vi "Labview online.vi"() -> ()   [LabVIEW 2019]
uses:
  <vilib>/sound2/lvsound2.llb/Sound Data Format.ctl
  <vilib>/sound2/lvsound2.llb/Sampling Mode.ctl
  <vilib>/sound2/lvsound2.llb/Sound Input Read (DBL).vi
  <vilib>/sound2/lvsound2.llb/Sound Output Write (DBL).vi
  <vilib>/Analysis/NI_AAL_SigProc.lvlib
  <vilib>/gmath/NI_Gmath.lvlib
panel:
  out "Envelope do Sinal":dynamicdata(graph)
  in  "stop":bool
  in  "Email":string
  in  "Gravar e Enviar":bool
  in  "Som de Saída":path
  in  "Terminar Medição":bool
  out "Número de Amostras Totais":dbl
  out "Taxa de Amostragem do Microfone (S/s)":dbl
  in  "Sound Format Input":T1={"sample rate (S/s)"=22050.0, "number of channels"=2, "bits per sample"=16}
  out "Ritmo Cardíaco Médio":dbl format="%0.2f"
  in  "Classificação do Ritmo Cardíaco":bool
  out "Taquicardia":bool
  out "Ritmo Cardíaco Normal":bool
  out "Bradicardia":bool
  in  "Continuar":bool
  out "Sinal Amplificado":waveform(dbl)[](graph)
  out "Sinal Amplificado e Filtrado":dynamicdata(graph)
  in  "Pulmões  ou Coração (pressionar)":bool
  in  "Controlador de Threshold":dbl(slide) scale=0.0..0.01
  out "Ritmo Cardíaco Instantaneo":dbl
  out "Offline Sound":dbl[](array[numeric])
  # "Estetoscópio Digital"
  # "Resultados"
  # "Configurações e Controlos"
  # "Parâmetros do Sinal de Som"
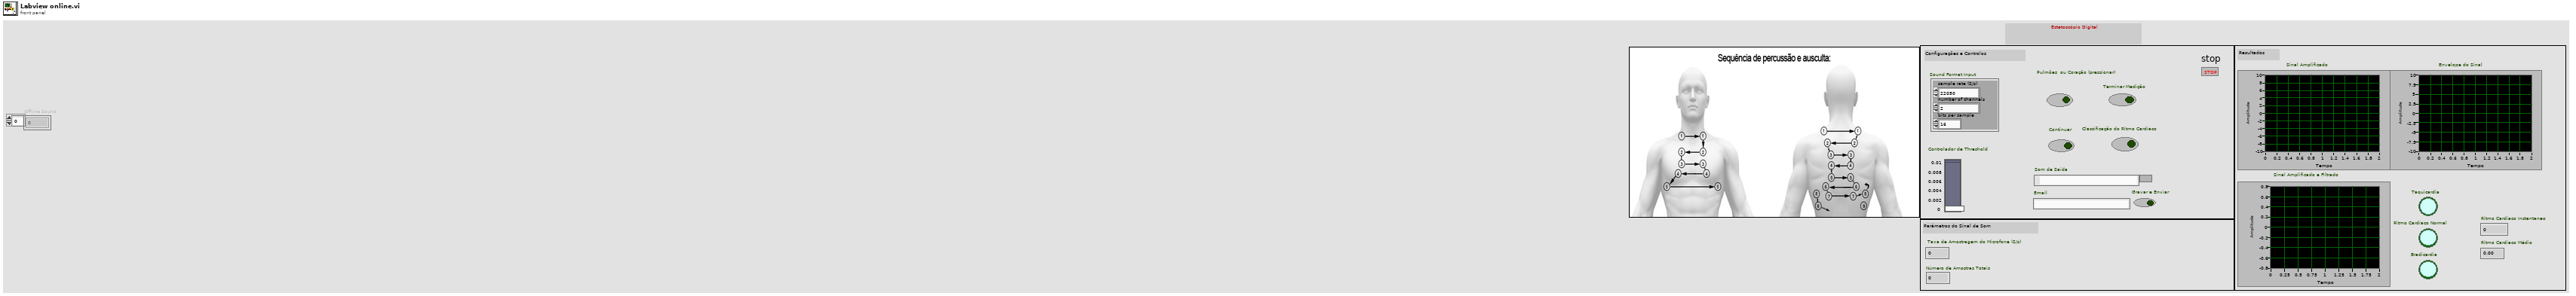
[diagram p1: front panel]
types:
  T1 = typedef "Sound Data Format.ctl" = cluster{"sample rate (S/s)":dbl, "number of channels":i32, "bits per sample":i32}
  T2 = typedef "Sampling Mode.ctl" = i32
  T3 = typedef "Sound Output Task ID.ctl" = u32
  T4 = typedef "Sound Input Task ID.ctl" = u32
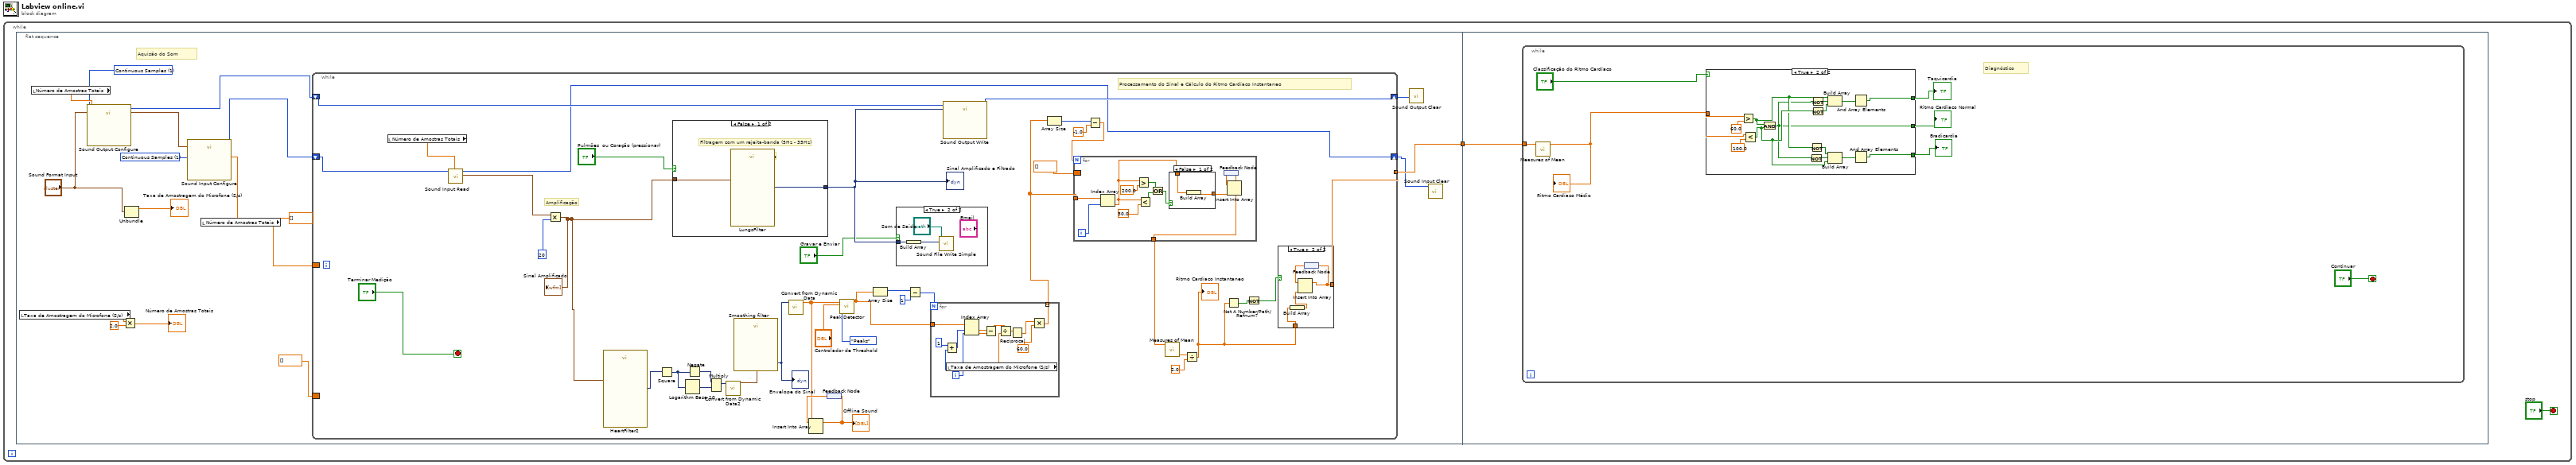
[diagram p0: block diagram]
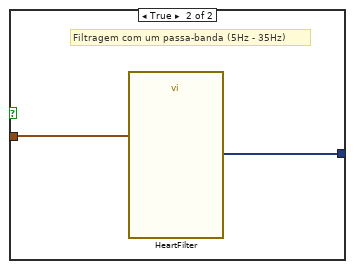
[diagram p5: hidden frame]
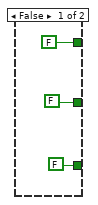
[diagram p6: hidden frame]
diagram:
  n1 = while {
    stop <- "stop" stop-if-true
    n2 = flat-sequence {
      tunnel: [w15] -> w2
      tunnel: w2 -> [w95]
      frame #0 {
        w6 = T2 1 items=["Finite Samples", "Continuous Samples"] ("sample mode")
        w14 = T2 1 items=["Finite Samples", "Continuous Samples"] ("sample mode")
        # "Aquisão do Som"
        n3 = local read "Taxa de Amostragem do Microfone (S/s)"() -> (w11:dbl)
        n4 = local read "Número de Amostras Totais"() -> (w8:dbl)
        n5 = call <vilib>:"Sound Output Configure.vi"("number of samples/ch"=w8, "sample mode"=w6, "sound format"="Sound Format Input") -> ("task ID"=w3:T3)  [unwired: 3 in, 5 out]
        n6 = Multiply(x=w11, y=2.0) -> (x*y=→"Número de Amostras Totais":dbl)
        n7 = Unbundle("Sound Format Input") -> ("sample rate (S/s)"=→"Taxa de Amostragem do Microfone (S/s)":dbl)  [unwired: 2 out]
        n8 = local read "Número de Amostras Totais"() -> (w7:dbl)
        n9 = call <vilib>:"Sound Input Configure.vi"("number of samples/ch"=w7, "sample mode"=w14, "sound format"="Sound Format Input") -> ("task ID"=w5:T4)  [unwired: 3 in, 5 out]
        n10 = while {
          shift-right: [w57] -> w16
          shift-left: w3 -> [w28]
          tunnel: [w44] -> w15
          border: dbl[] [] -> [_]
          border: dbl[] [] -> [_]
          shift-right: [w24] -> w4
          shift-left: w5 -> [w26]
          stop <- "Terminar Medição" stop-if-true
          # "Processamento do Sinal e Cálculo do Ritmo Cardíaco Instantaneo"
          # "Filter Stage"
          # "Amplificação"
          n11 = local read "Número de Amostras Totais"() -> (w27:dbl)
          n12 = call-poly <vilib>:"Sound Input Read.vi"("number of samples/ch"=w27, "task ID"=w26) -> ("data"=w25:waveform(dbl)[], "task ID out"=w24:T4)  [unwired: 2 in, 6 out]
          n13 = Multiply(x=w25, y=20) -> (x*y=w20:waveform(dbl)[])
          "Sinal Amplificado" <- w20
          n14 = call "HeartFilter2"("Signal"=w20) -> ("Filtered Signal"=w35:dynamicdata)  [unwired: 9 in, 1 out]
          n15 = Square(x=w35) -> (x^2=w38:dynamicdata)
          n16 = case shown="False" "Pulmões  ou Coração (pressionar)" {
            tunnel: w20 -> [w92 w94]
            tunnel: [w91 w93] -> w23
            frame False {
              # "Filtragem com um rejeita-banda (5Hz - 35Hz)"
              n17 = call "LungsFilter"("Signal"=w92) -> ("Filtered Signal"=w91:dynamicdata)  [unwired: 9 in, 1 out]
            }
            frame True {
              # "Filtragem com um passa-banda (5Hz - 35Hz)"
              n18 = call "HeartFilter"("Signal"=w94) -> ("Filtered Signal"=w93:dynamicdata)  [unwired: 9 in, 1 out]
            }
          }
          "Sinal Amplificado e Filtrado" <- w23
          n19 = Logarithm Base 10(1:w38) -> (0:w40:dynamicdata)
          n20 = Negate(x=w38) -> (-x=w39:dynamicdata)
          n21 = Multiply(1:w40, 2:w39) -> (0:w36:dynamicdata)  [unwired: 1 in, 1 out]
          n22 = call "Convert from Dynamic Data2"("Dynamic Data Type"=w36) -> ("Waveform"=w37:waveform(dbl))  [unwired: 3 in]
          n23 = call "Smoothing filter"("Signal"=w37) -> ("Filtered Signal"=w19:dynamicdata)  [unwired: 9 in, 1 out]
          "Envelope do Sinal" <- w19
          n24 = call "Convert from Dynamic Data"("Dynamic Data Type"=w19) -> ("Array"=w32:dbl[])  [unwired: 3 in]
          n25 = feedback #1() -> (w41:dbl[])
          n26 = Insert Into Array(array=w41, new element=w32) -> (w34:dbl[])  [unwired: 1 in]
          "Offline Sound" <- w34
          n27 = feedback-in #1(w34) -> ()
          n28 = call <vilib>:"Peak Detector.vi"("peaks/valleys"=enum32{"Peaks", "Valleys"}."Peaks", "threshold"="Controlador de Threshold", "X"=w32) -> ("Locations"=w51:dbl[])  [unwired: 4 in, 4 out]
          n29 = Array Size(array=w51) -> (size(s)=w52:i32)
          n30 = case shown="True" "Gravar e Enviar" {
            tunnel: w23 -> [_ w60]
            frame False {
            }
            frame True {
              n31 = Build Array(w60) -> (w61:dynamicdata[])
              n32 = call <vilib>:"Sound File Write Simple.vi"("data"=w61, "path"="Som de Saída") -> ()  [unwired: 8 in, 2 out]
            }
          }
          n33 = Subtract(x=w52, y=1) -> (x-y=w53:i32)
          n34 = for {
            N: w53 -> [_]
            tunnel: w51 -> [w88]
            tunnel: [w79] -> w46 mode=indexing
            i -> [w83]
            n35 = Add(x=1 ("y"), y=w83) -> (x+y=w84:i32)
            n36 = local read "Taxa de Amostragem do Microfone (S/s)"() -> (w80:dbl)
            n37 = Index Array(array=w88, index #1=w84, index #2=w83) -> (element #1=w87:dbl, element #2=w82:dbl)
            n38 = Subtract(x=w87, y=w82) -> (x-y=w81:dbl)
            n39 = Divide(x=w81, y=w80) -> (x/y=w86:dbl)
            n40 = Reciprocal(x=w86) -> (1/x=w90:dbl)
            n41 = Multiply(x=w90, y=60.0) -> (x*y=w79:dbl)
          }
          n42 = call-poly <vilib>:"Sound Output Write.vi"("data"=w23, "task ID"=w28) -> ("task ID out"=w57:T3)  [unwired: 2 in, 7 out]
          n43 = Array Size(array=w46) -> (size(s)=w49:i32)
          n44 = Subtract(x=w49, y=-1.0) -> (x-y=w48:dbl)
          n45 = for {
            N: w48 -> [_]
            tunnel: w46 -> [w70]
            tunnel: [w66] -> w45
            border: dbl[] [] -> [_]
            i -> [w71]
            n46 = Index Array(array=w70, index=w71) -> (element=w69:dbl)
            n47 = Greater?(x=w69, y=200.0) -> (0:w74:bool)
            n48 = Less?(x=w69, y=30.0) -> (x < y?=w73:bool)
            n49 = Or(x=w74, y=w73) -> (x .or. y?=w72:bool)
            n50 = case shown="False" w72 {
              tunnel: w69 -> [w78 _]
              tunnel: [w77 _] -> w68
              frame False {
                n51 = Build Array(w78) -> (w77:dbl[])
              }
              frame True {
              }
            }
            n52 = feedback #2() -> (w67:dbl[])
            n53 = Insert Into Array(array=w67, new element=w68) -> (w66:dbl[])  [unwired: 1 in]
            n54 = feedback-in #2(w66) -> ()
          }
          n55 = call <vilib>:"Measures of Mean.vi"("x array"=w45) -> ("mean value"=w31:dbl)  [unwired: 9 in, 1 out]
          n56 = Divide(x=w31, y=2.0) -> (x/y=w30:dbl)
          "Ritmo Cardíaco Instantaneo" <- w30
          n57 = Not A Number/Path/Refnum?(number/path/refnum=w30) -> (NaN/Path/Refnum?=w43:bool)
          n58 = Not(x=w43) -> (.not. x?=w42:bool)
          n59 = case shown="True" w42 {
            tunnel: [_ w64] -> w44
            tunnel: w30 -> [_ w63]
            frame False {
            }
            frame True {
              n60 = Build Array(w63) -> (w62:dbl[])
              n61 = feedback #3() -> (w65:dbl[])
              n62 = Insert Into Array(array=w65, new element=w62) -> (w64:dbl[])  [unwired: 1 in]
              n63 = feedback-in #3(w64) -> ()
            }
          }
        }
        n64 = call <vilib>:"Sound Output Clear.vi"("task ID"=w16) -> ()  [unwired: 10 in, 1 out]
        n65 = call <vilib>:"Sound Input Clear.vi"("task ID"=w4) -> ()  [unwired: 1 in, 10 out]
      }
      frame #1 {
        n66 = while {
          tunnel: w95 -> [w99]
          stop <- "Continuar" stop-if-true
          # "Diagnóstico"
          n67 = call <vilib>:"Measures of Mean.vi"("x array"=w99) -> ("mean value"=w97:dbl)  [unwired: 9 in, 1 out]
          "Ritmo Cardíaco Médio" <- w97
          n68 = case shown="True" "Classificação do Ritmo Cardíaco" {
            tunnel: w97 -> [_ w117]
            tunnel: [FALSE w108] -> w102
            tunnel: [FALSE w107] -> w101
            tunnel: [FALSE w106] -> w100
            frame False {
            }
            frame True {
              n69 = Greater?(x=w117, y=60.0) -> (0:w110:bool)
              n70 = Less?(x=w117, y=100.0) -> (x < y?=w112:bool)
              n71 = And(x=w110, y=w112) -> (x .and. y?=w107:bool)
              n72 = Not(x=w107) -> (.not. x?=w113:bool)
              n73 = Not(x=w110) -> (.not. x?=w111:bool)
              n74 = Not(x=w107) -> (.not. x?=w115:bool)
              n75 = Not(x=w112) -> (.not. x?=w114:bool)
              n76 = Build Array(w110, w115, w114) -> (w116:bool[])
              n77 = Build Array(w111, w113, w112) -> (w109:bool[])
              n78 = And Array Elements(Boolean array=w116) -> (logical AND=w106:bool)
              n79 = And Array Elements(Boolean array=w109) -> (logical AND=w108:bool)
            }
          }
          "Taquicardia" <- w100
          "Ritmo Cardíaco Normal" <- w101
          "Bradicardia" <- w102
        }
      }
    }
  }
